vi "Outgoing Sub-Section Page.vi"(8 "error in (no error)":errorcluster, 11 "Node Ptr":T4 format="%.0x") -> (0 "error out":errorcluster)   [LabVIEW 2023, in "Protection and Counter Addon System Explorer.lvlib"]
uses:
  Protection and Counter Addon System Explorer.lvlib
  <vilib>/NI VeriStand/Custom Device API/Custom Device Item Ref.ctl
  Types/Event Trigger Type.ctl
  <vilib>/NI VeriStand/UI Controls/Single Node Browser/Net Event Data.ctl
  <vilib>/NI VeriStand/UI Controls/Single Node Browser/Net Event.ctl
  Addon Shared/SubVIs/GUID Lookup.vi
  <vilib>/NI VeriStand/Custom Device API/Get Item Property (U32).vi
  <vilib>/NI VeriStand/Custom Device API/Set Item Property (U32).vi
  <vilib>/NI VeriStand/Custom Device API/Get Item Property (Dependent Node Pointer).vi
  <vilib>/NI VeriStand/Custom Device API/Set Item Property (Dependent Node Pointer).vi
  <vilib>/NI VeriStand/Custom Device API/Custom Device API.lvlib
  Addon Shared/Protection and Counter Addon Shared.lvlib
  SubModules/Frame-Protection-Support/Source/System Explorer/Protection and Counter Support System Explorer.lvlib
  <vilib>/NI VeriStand/UI Controls/Single Node Browser/NI_VS UI Single Node Browser.lvlib
  NationalInstruments.VeriStand.SystemStorageUI
panel:
  in  "Specific Header 2":T1={"Transmit Trigger Batch Settings"="Transmit Trigger Settings"}
  in  "OK2":bool
  in  "Transmit Trigger":T2
  in  "Trigger":refnum<k24>(container)
  in  "OK1":bool
  in  "Start Time Offset (ms)":u32
  out "Version":string
  in  "SHDocVw.IWebBrowser":refnum<k7>(container)
  in  "Specific Header":T3={"Start Time Offset Batch Settings"="Start Time Offset Settings"}
  in  "General Header":cluster{"Section Name":string}={"Section Name"="General Custom Device Settings"}
  in  "Description":string
  in  "Name":string
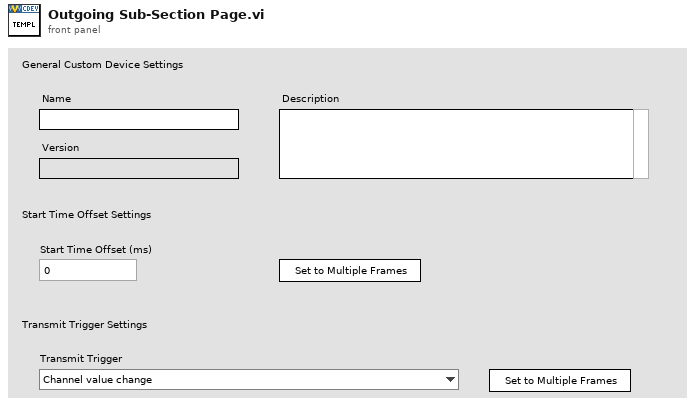
[diagram p1: front panel]
types:
  T1 = cluster{"Transmit Trigger Batch Settings":string}
  T2 = typedef "Protection and Counter Addon System Explorer.lvlib/Event Trigger Type.ctl" = enum16{"Channel value change", "Trigger channel (not zero)", "Channel value change or trigger channel (not zero)", "Trigger channel (any value change)", "Channel value change or trigger channel (any value change)"}
  T3 = cluster{"Start Time Offset Batch Settings":string}
  T4 = typedef "Custom Device API.lvlib/Custom Device Item Ref.ctl" = u64
  T5 = typedef "Custom Device API.lvlib/Custom Device Item Info.ctl" = cluster{"Name":string, "Is Channel":bool, "GUID":string, "Is Waveform":bool}
  T6 = typedef "NI_VS UI Single Node Browser.lvlib/Single Node Browser Ref.ctl" = refnum<k24>
  T7 = typedef "NI_VS UI Single Node Browser.lvlib/Callback Type.ctl" = cluster{"Net Callbacks":refnum<k27>[], "Event":refnum<user-event>}
  T8 = typedef "Custom Device API.lvlib/Custom Device Commands.ctl" = enum16{"Default", "Item renamed", "Shutdown", "Dynamic button pressed"}
  T9 = typedef "Protection and Counter Support System Explorer.lvlib/Protection Signal Linked Channel.ctl" = cluster{"Node Ref":T4}
  T10 = typedef "Protection and Counter Addon System Explorer.lvlib/Frame Settings.ctl" = cluster{"ID":u32, "Disable Transmission":bool, "Disable Transmission Ref":T4, "Transmit Trigger":T2, "Transmit Trigger Ref":T4, "Start Time Offset (ms)":u32, "Tx Control.Disable Tx Ref":T4, "Tx Control.Override Period Ref":T4, "Tx Control.Override Period Value Ref":T4}
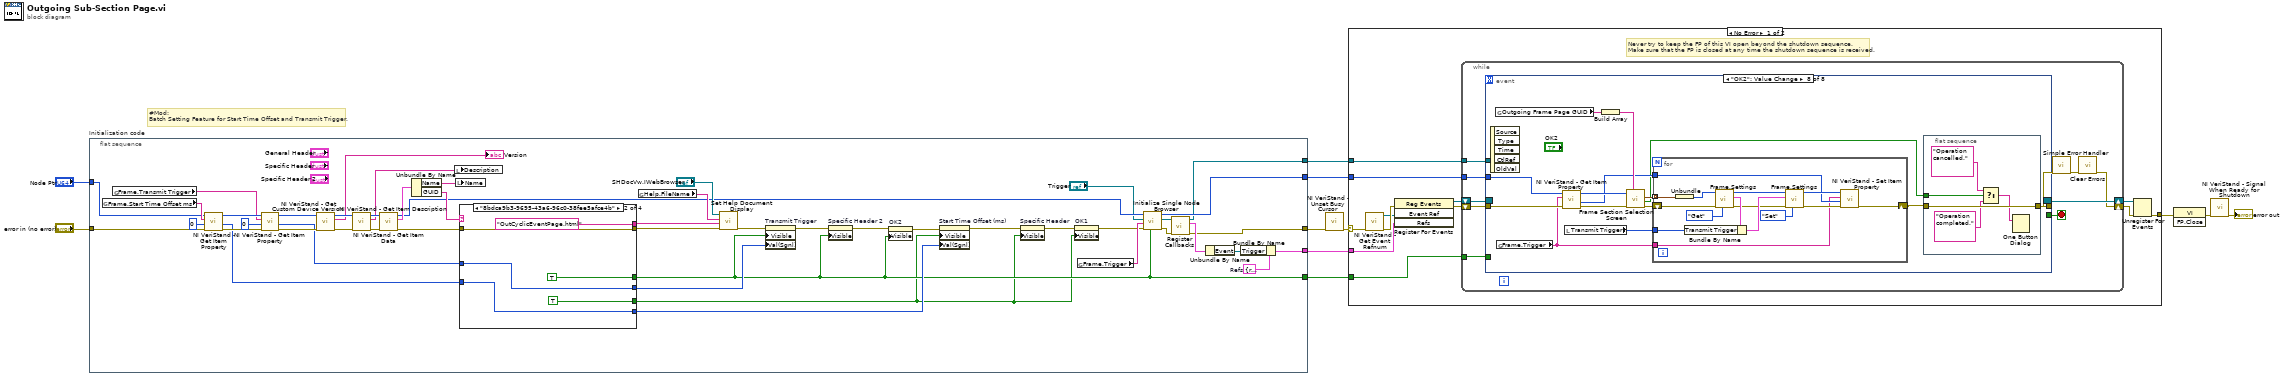
[diagram p0: block diagram]
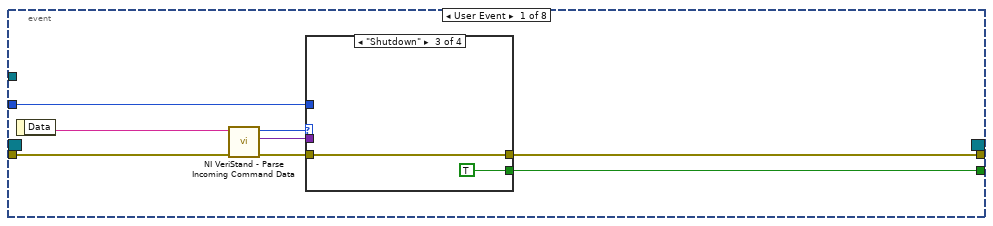
[diagram p2: hidden frame]
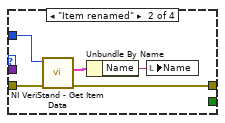
[diagram p4: hidden frame]
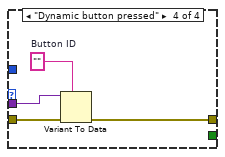
[diagram p5: hidden frame]
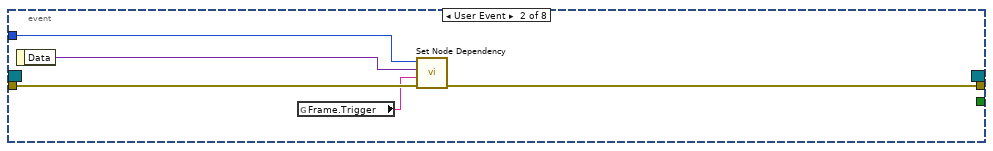
[diagram p6: hidden frame]
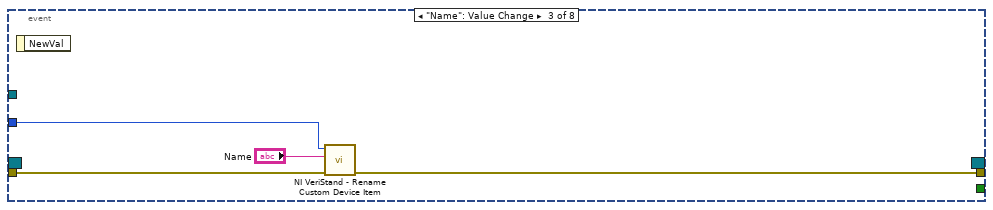
[diagram p7: hidden frame]
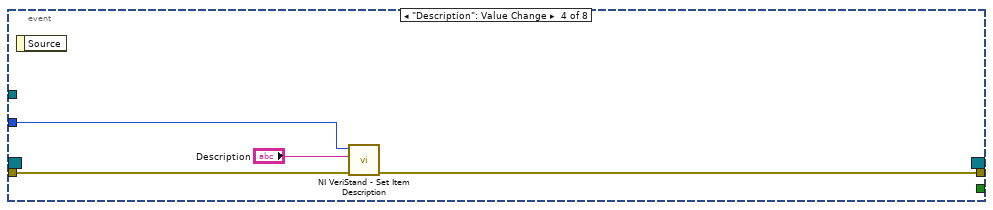
[diagram p8: hidden frame]
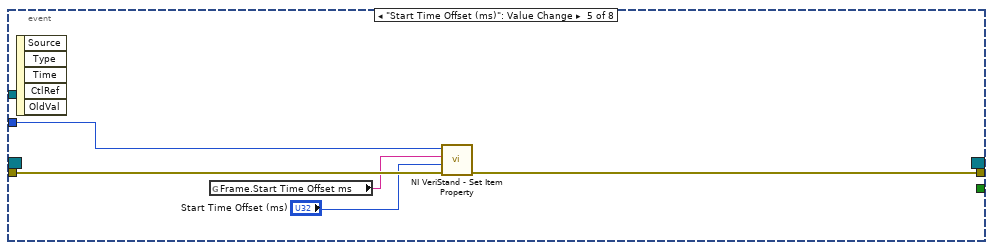
[diagram p9: hidden frame]
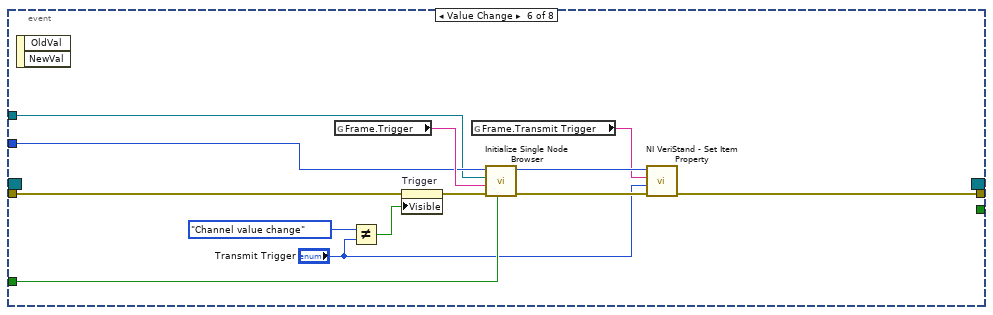
[diagram p10: hidden frame]
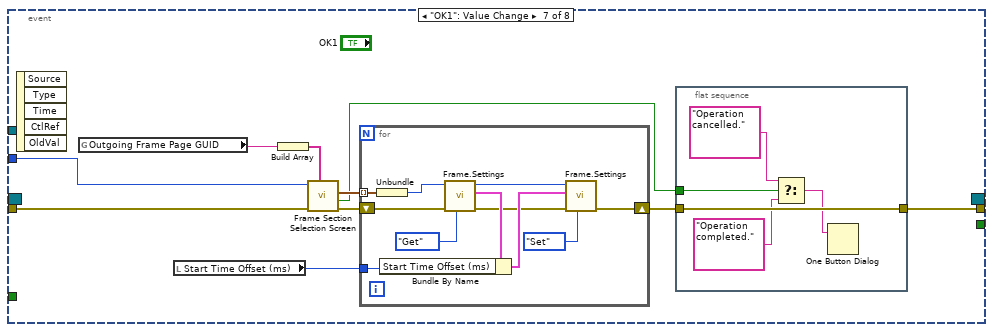
[diagram p11: hidden frame]
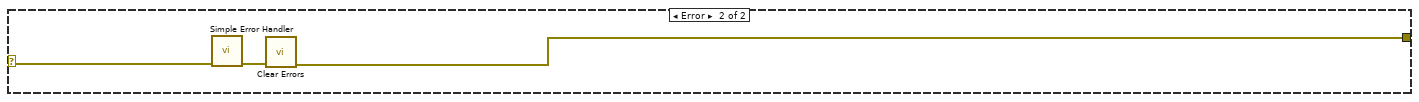
[diagram p12: hidden frame]
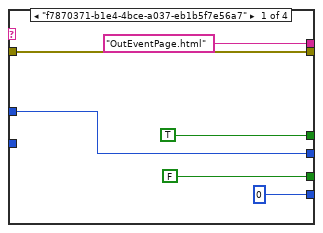
[diagram p13: hidden frame]
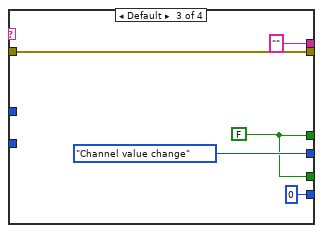
[diagram p14: hidden frame]
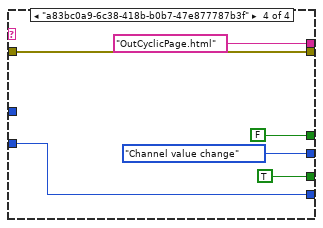
[diagram p15: hidden frame]
diagram:
  # "#Mod:\nBatch Setting Feature for Start Time Offset and Transmit Trigger."
  n1 = flat-sequence "Initialization code" {
    tunnel: "error in (no error)" -> [w12]
    tunnel: "Node Ptr" -> [w13]
    tunnel: [w34] -> w7
    tunnel: [w35] -> w4
    tunnel: [w31] -> w3
    tunnel: [w30] -> w2
    tunnel: [w28] -> w1
    frame #0 {
      w33 = cluster{"Trigger":refnum<user-event>} {"Trigger"=refnum}  # Refs
      n2 = global read "GUID Lookup.vi" "Frame.Start Time Offset ms"() -> (w16:string)
      n3 = global read "GUID Lookup.vi" "Frame.Transmit Trigger"() -> (w15:string)
      n4 = call-poly <vilib>:"NI VeriStand - Get Item Property.vi"("error in (no error)"=w12, "Default Value"=u32 0, "Property Name"=w16, "Item Ref in"=w13) -> ("error out"=w19:errorcluster, "Value"=w14:u32, "Item Ref out"=w21:T4)  [unwired: 4 in, 1 out]
      n5 = call-poly <vilib>:"NI VeriStand - Get Item Property.vi"("error in (no error)"=w19, "Default Value"=u32 0, "Property Name"=w15, "Item Ref in"=w21) -> ("error out"=w18:errorcluster, "Value"=w17:u32, "Item Ref out"=w20:T4)  [unwired: 4 in, 1 out]
      n6 = call <vilib>:"NI VeriStand - Get Custom Device Version.vi"("error in (no error)"=w18, "Device Ref in"=w20) -> ("error out"=w57:errorcluster, "Value"=→"Version":string, "Device Ref out"=w56:T4)  [unwired: 7 in]
      n7 = call <vilib>:"NI VeriStand - Get Item Description.vi"("error in (no error)"=w57, "Item Ref in"=w56) -> ("error out"=w59:errorcluster, "Description"=w53:string, "Item Ref out"=w60:T4)  [unwired: 7 out]
      n8 = call <vilib>:"NI VeriStand - Get Item Data.vi"("error in (no error)"=w59, "Item Ref in"=w60) -> ("error out"=w51:errorcluster, "Item Info"=w58:T5, "Item Ref out"=w37:T4)  [unwired: 7 out]
      n9 = Unbundle By Name(w58) -> ("Name"=w54:string, "GUID"=w50:string)
      n10 = local write "Description"(w53) -> ()
      n11 = local write "Name"(w54) -> ()
      n12 = case shown="\"8bdca9b3-9695-43a6-96c0-38fee5afce4b\"" w50 {
        tunnel: ["OutEventPage.html" ("HTML File") "OutCyclicEventPage.html" ("HTML File") "" ("HTML File") "OutCyclicPage.html" ("HTML File")] -> w47
        tunnel: w51 -> [w65 w71 w76 w82]
        tunnel: [w65 w71 w76 w82] -> w49
        tunnel: [TRUE TRUE w74 FALSE] -> w28
        tunnel: [w63 w69 Event_Trigger_Type."Channel value change" ("y") Event_Trigger_Type."Channel value change" ("y")] -> w44
        tunnel: w17 -> [w63 w69 _ _]
        tunnel: w14 -> [_ w67 _ w79]
        tunnel: [u16 0 ("Start Time Offset (ms)") w67 u16 0 ("Start Time Offset (ms)") w79] -> w43
        tunnel: [FALSE TRUE w74 TRUE] -> w25
        frame "f7870371-b1e4-4bce-a037-eb1b5f7e56a7" {
        }
        frame "8bdca9b3-9695-43a6-96c0-38fee5afce4b" {
        }
        frame Default {
          w74 = FALSE
        }
        frame "a83bc0a9-6c38-418b-b0b7-47e877787b3f" {
        }
      }
      n13 = global read "GUID Lookup.vi" "Help.FileName"() -> (w52:string)
      n14 = call "Set Help Document Display.vi"("error in (no error)"=w49, "HTML File"=w47, "Main CHM File"=w52, "SHDocVw.IWebBrowser2"="SHDocVw.IWebBrowser") -> ("error out"=w45:errorcluster)  [unwired: 7 in]
      n15 = property on="Transmit Trigger" class="Enum (strict)"(error in=w45, "Visible"=w28, "Val(Sgnl)"=w44) -> (error out=w46:errorcluster)  [unwired: 1 in, 1 out]
      n16 = property on="Specific Header 2" class="Clust (strict)"(error in=w46, "Visible"=w28) -> (error out=w29:errorcluster)  [unwired: 1 in, 1 out]
      n17 = property on="OK2" class="Bool"(error in=w29, "Visible"=w28) -> (error out=w27:errorcluster)  [unwired: 1 in, 1 out]
      n18 = property on="Start Time Offset (ms)" class="DigNum (strict)"(error in=w27, "Visible"=w25, "Val(Sgnl)"=w43) -> (error out=w42:errorcluster)  [unwired: 1 in, 1 out]
      n19 = property on="Specific Header" class="Clust (strict)"(error in=w42, "Visible"=w25) -> (error out=w26:errorcluster)  [unwired: 1 in, 1 out]
      n20 = property on="OK1" class="Bool"(error in=w26, "Visible"=w25) -> (error out=w24:errorcluster)  [unwired: 1 in, 1 out]
      n21 = global read "GUID Lookup.vi" "Frame.Trigger"() -> (w38:string)
      n22 = call "Initialize Single Node Browser.vi"("Use Channel?"=w28, "error in (no error)"=w24, "NodeName"=w38, "Browser Ref 2"="Trigger", "Item Ref in"=w37) -> ("error out"=w39:errorcluster, "Browser Ref"=w40:T6, "Item Ref out"=w35:T4)  [unwired: 4 in]
      n23 = call <vilib>:"Register Callbacks.vi"("error in (no error)"=w39, "Single Node Browser"=w40) -> ("error out"=w34:errorcluster, "Callbacks"=w41:T7, "Single Node Browser dup"=w30:T6)  [unwired: 7 in]
      n24 = Unbundle By Name(w41) -> ("Event"=w32:refnum<user-event>)
      n25 = Bundle By Name(cluster=w33, "Trigger"=w32) -> (w31:cluster{"Trigger":refnum<user-event>})
    }
  }
  n26 = call <vilib>:"NI VeriStand - Unset Busy Cursor.vi"("error in (no error)"=w7) -> ("error out"=w6:errorcluster)  [unwired: 10 out]
  n27 = case shown="No Error" w6 {
    selector: w6 -> [w87 w219]
    tunnel: [w92 w217] -> w11
    tunnel: w4 -> [w88 _]
    tunnel: w3 -> [w86 _]
    tunnel: w2 -> [w85 _]
    tunnel: w1 -> [w84 _]
    frame No Error {
      # "Never try to keep the FP of this VI open beyond the shutdown sequence.\nMake sure that the FP is closed at any time the shutdown sequence is received."
      n28 = call <vilib>:"NI VeriStand - Get Event Refnum.vi"("error in (no error)"=w87) -> ("error out"=w95:errorcluster, "Event Ref"=w91:refnum<user-event>)  [unwired: 9 out]
      n29 = register-events(error in=w95, w91, w86) -> (reference out=w89:refnum<event-registration>, error out=w90:errorcluster)  [unwired: 1 in]
      n30 = while {
        tunnel: w88 -> [w101]
        shift-right: [w98] -> w93
        shift-left: w90 -> [w104]
        shift-right: [w105] -> w94
        shift-left: w89 -> [w103]
        tunnel: w85 -> [w97]
        tunnel: w84 -> [w96]
        stop <- w102 stop-if-true
        n31 = event shown="[7] \"OK2\": Value Change" {
          selector: w103 -> [_ _ _ _ _ _ _ _]
          dyn-events: [_ _ _ _ _ _ _ _] -> w105
          timeout: _ -> [_ _ _ _ _ _ _ _]
          tunnel: w104 -> [w113 w130 w134 w137 w142 w151 w166 w191]
          tunnel: [w109 _ _ _ _ _ _ _] -> w102
          tunnel: [w108 w126 w133 w136 w143 w144 w158 w184] -> w100
          tunnel: w101 -> [w107 w128 w132 w138 w140 w152 w164 w190]
          tunnel: w97 -> [_ _ _ _ _ w150 _ _]
          tunnel: w96 -> [_ _ _ _ _ w149 _ _]
          event User Event {
            n32 = event-data() -> ("Data"=w112:string)  [unwired: 1 out]
            n33 = call <vilib>:"NI VeriStand - Parse Incoming Command Data.vi"("error in (no error)"=w113, "Incoming data"=w112) -> ("error out"=w111:errorcluster, "Outgoing data"=w106:variant, "Action"=w110:T8)  [unwired: 7 out]
            n34 = case shown="\"Shutdown\"" w110 {
              tunnel: w111 -> [w114 w119 w120 w125]
              tunnel: [_ _ TRUE _] -> w109
              tunnel: [w114 w116 w120 w122] -> w108
              tunnel: w107 -> [_ w118 _ _]
              tunnel: w106 -> [_ _ _ w124]
              frame "Default", Default {
              }
              frame "Item renamed" {
                n35 = call <vilib>:"NI VeriStand - Get Item Data.vi"("error in (no error)"=w119, "Item Ref in"=w118) -> ("error out"=w116:errorcluster, "Item Info"=w117:T5)  [unwired: 8 out]
                n36 = Unbundle By Name(w117) -> ("Name"=w115:string)
                n37 = local write "Name"(w115) -> ()
              }
              frame "Shutdown" {
              }
              frame "Dynamic button pressed" {
                w123 = ""  # Button ID
                n38 = Variant To Data(error in=w125, type=w123, Variant=w124) -> (error out=w122:errorcluster)  [unwired: 1 out]
              }
            }
          }
          event User Event {
            n39 = event-data() -> ("Data"=w129:variant)  [unwired: 1 out]
            n40 = global read "GUID Lookup.vi" "Frame.Trigger"() -> (w127:string)
            n41 = call "Set Node Dependency.vi"("error in (no error)"=w130, "NodeName"=w127, "Data"=w129, "Item Ref in"=w128) -> ("error out"=w126:errorcluster)  [unwired: 6 in, 1 out]
          }
          event "Name": Value Change {
            n42 = event-data() -> ()  [unwired: 2 out]
            n43 = call <vilib>:"NI VeriStand - Rename Custom Device Item.vi"("error in (no error)"=w134, "New Name"="Name", "Item Ref in"=w132) -> ("error out"=w133:errorcluster)  [unwired: 1 in, 7 out]
          }
          event "Description": Value Change {
            n44 = event-data() -> ()  [unwired: 2 out]
            n45 = call <vilib>:"NI VeriStand - Set Item Description.vi"("error in (no error)"=w137, "Description"="Description", "Item Ref in"=w138) -> ("error out"=w136:errorcluster)  [unwired: 8 out]
          }
          event "Start Time Offset (ms)": Value Change {
            n46 = event-data() -> ()  [unwired: 6 out]
            n47 = global read "GUID Lookup.vi" "Frame.Start Time Offset ms"() -> (w139:string)
            n48 = call-poly <vilib>:"NI VeriStand - Set Item Property.vi"("error in (no error)"=w142, "Value"="Start Time Offset (ms)", "Property Name"=w139, "Item Ref in"=w140) -> ("error out"=w143:errorcluster)  [unwired: 5 in, 2 out]
          }
          event Value Change {
            n49 = event-data() -> ()  [unwired: 3 out]
            n50 = global read "GUID Lookup.vi" "Frame.Trigger"() -> (w153:string)
            n51 = Not Equal?(x=Event_Trigger_Type."Channel value change" ("y"), y="Transmit Trigger") -> (x != y?=w154:bool)
            n52 = property on="Trigger" class="AXCont"(error in=w151, "Visible"=w154) -> (error out=w156:errorcluster)  [unwired: 1 in, 1 out]
            n53 = global read "GUID Lookup.vi" "Frame.Transmit Trigger"() -> (w146:string)
            n54 = call "Initialize Single Node Browser.vi"("Use Channel?"=w149, "error in (no error)"=w156, "NodeName"=w153, "Browser Ref 2"=w150, "Item Ref in"=w152) -> ("error out"=w147:errorcluster, "Item Ref out"=w148:T4)  [unwired: 4 in, 1 out]
            n55 = call-poly <vilib>:"NI VeriStand - Set Item Property.vi"("error in (no error)"=w147, "Value"="Transmit Trigger", "Property Name"=w146, "Item Ref in"=w148) -> ("error out"=w144:errorcluster)  [unwired: 5 in, 2 out]
          }
          event "OK1": Value Change {
            n56 = event-data() -> ()  [unwired: 6 out]
            n57 = global read "GUID Lookup.vi" "Outgoing Frame Page GUID"() -> (w163:string)
            n58 = local read "Start Time Offset (ms)"() -> (w160:u32)
            n59 = Build Array(w163) -> (w165:string[])
            n60 = call "Frame Section Selection Screen.vi"("guids"=w165, "error in"=w166, "Parent Ref"=w164) -> ("error out"=w161:errorcluster, "Cancelled?"=w157:bool, "Output Selections"=w162:T9[])  [unwired: 5 in, 1 out]
            n61 = for {
              tunnel: w162 -> [w182] mode=indexing
              tunnel: w160 -> [w173]
              shift-right: [w172] -> w159
              shift-left: w161 -> [w175]
              n62 = Unbundle(w182) -> ("Node Ref"=w174:T4)
              n63 = call "Frame.Settings.vi"("Action"=enum8{"Get", "Set"}."Get", "error in (no error)"=w175, "Item Ref in"=w174) -> ("error out"=w178:errorcluster, "Frame.Settings"=w180:T10, "Item Ref out"=w179:T4)  [unwired: 6 in]
              n64 = Bundle By Name(cluster=w180, "Start Time Offset (ms)"=w173) -> (w181:T10)
              n65 = call "Frame.Settings.vi"("Action"=enum8{"Get", "Set"}."Set", "error in (no error)"=w178, "Frame.Settings"=w181, "Item Ref in"=w179) -> ("error out"=w172:errorcluster)  [unwired: 5 in, 2 out]
            }
            n66 = flat-sequence {
              tunnel: w159 -> [w171]
              tunnel: [w171] -> w158
              tunnel: w157 -> [w170]
              frame #0 {
                n67 = Select(t="Operation cancelled." ("message"), s=w170, f="Operation completed." ("message")) -> (s? t:f=w167:string)
                n68 = One Button Dialog(message=w167) -> ()  [unwired: 1 in, 1 out]
              }
            }
          }
          event "OK2": Value Change {
            n69 = event-data() -> ()  [unwired: 6 out]
            n70 = global read "GUID Lookup.vi" "Outgoing Frame Page GUID"() -> (w195:string)
            n71 = global read "GUID Lookup.vi" "Frame.Trigger"() -> (w186:string)
            n72 = call-poly <vilib>:"NI VeriStand - Get Item Property.vi"("error in (no error)"=w191, "Property Name"=w186, "Item Ref in"=w190) -> ("error out"=w188:errorcluster, "Dependent Node Ref"=w187:T4, "Item Ref out"=w189:T4)  [unwired: 5 in, 1 out]
            n73 = local read "Transmit Trigger"() -> (w192:T2)
            n74 = Build Array(w195) -> (w196:string[])
            n75 = call "Frame Section Selection Screen.vi"("guids"=w196, "error in"=w188, "Parent Ref"=w189) -> ("error out"=w193:errorcluster, "Cancelled?"=w183:bool, "Output Selections"=w194:T9[])  [unwired: 5 in, 1 out]
            n76 = for {
              tunnel: w194 -> [w216] mode=indexing
              tunnel: w192 -> [w207]
              shift-right: [w205] -> w185
              shift-left: w193 -> [w209]
              tunnel: w187 -> [w203]
              tunnel: w186 -> [w202]
              n77 = Unbundle(w216) -> ("Node Ref"=w208:T4)
              n78 = call "Frame.Settings.vi"("Action"=enum8{"Get", "Set"}."Get", "error in (no error)"=w209, "Item Ref in"=w208) -> ("error out"=w212:errorcluster, "Frame.Settings"=w214:T10, "Item Ref out"=w213:T4)  [unwired: 6 in]
              n79 = Bundle By Name(cluster=w214, "Transmit Trigger"=w207) -> (w215:T10)
              n80 = call "Frame.Settings.vi"("Action"=enum8{"Get", "Set"}."Set", "error in (no error)"=w212, "Frame.Settings"=w215, "Item Ref in"=w213) -> ("error out"=w206:errorcluster, "Item Ref out"=w204:T4)  [unwired: 5 in, 1 out]
              n81 = call-poly <vilib>:"NI VeriStand - Set Item Property.vi"("error in (no error)"=w206, "Dependent Node Ref"=w203, "Property Name"=w202, "Item Ref in"=w204) -> ("error out"=w205:errorcluster)  [unwired: 5 in, 2 out]
            }
            n82 = flat-sequence {
              tunnel: w185 -> [w201]
              tunnel: [w201] -> w184
              tunnel: w183 -> [w200]
              frame #0 {
                n83 = Select(t="Operation cancelled." ("message"), s=w200, f="Operation completed." ("message")) -> (s? t:f=w197:string)
                n84 = One Button Dialog(message=w197) -> ()  [unwired: 1 in, 1 out]
              }
            }
          }
        }
        n85 = call <vilib>:"Simple Error Handler.vi"("error in (no error)"=w100) -> ("error out"=w99:errorcluster)  [unwired: 1 in, 7 out]
        n86 = call <vilib>:"Clear Errors.vi"("error in (no error)"=w99) -> ("error out"=w98:errorcluster)  [unwired: 1 in, 5 out]
      }
      n87 = Unregister For Events(event registration refnum=w94, error in=w93) -> (error out=w92:errorcluster)
    }
    frame Error {
      n88 = call <vilib>:"Simple Error Handler.vi"("error in (no error)"=w219) -> ("error out"=w218:errorcluster)  [unwired: 1 in, 7 out]
      n89 = call <vilib>:"Clear Errors.vi"("error in (no error)"=w218) -> ("error out"=w217:errorcluster)  [unwired: 1 in, 5 out]
    }
  }
  n90 = invoke class="VI" method="FP.Close"(error in=w11) -> (error out=w10:errorcluster)  [unwired: 2 in, 2 out]
  n91 = call <vilib>:"NI VeriStand - Signal When Ready for Shutdown.vi"("error in (no error)"=w10) -> ("error out"=→"error out":errorcluster)  [unwired: 10 out]
